vi "small_cap_hod_momentum.vi"() -> ()   [LabVIEW 2023]
panel:
  in  "MCLB":i32(listbox)
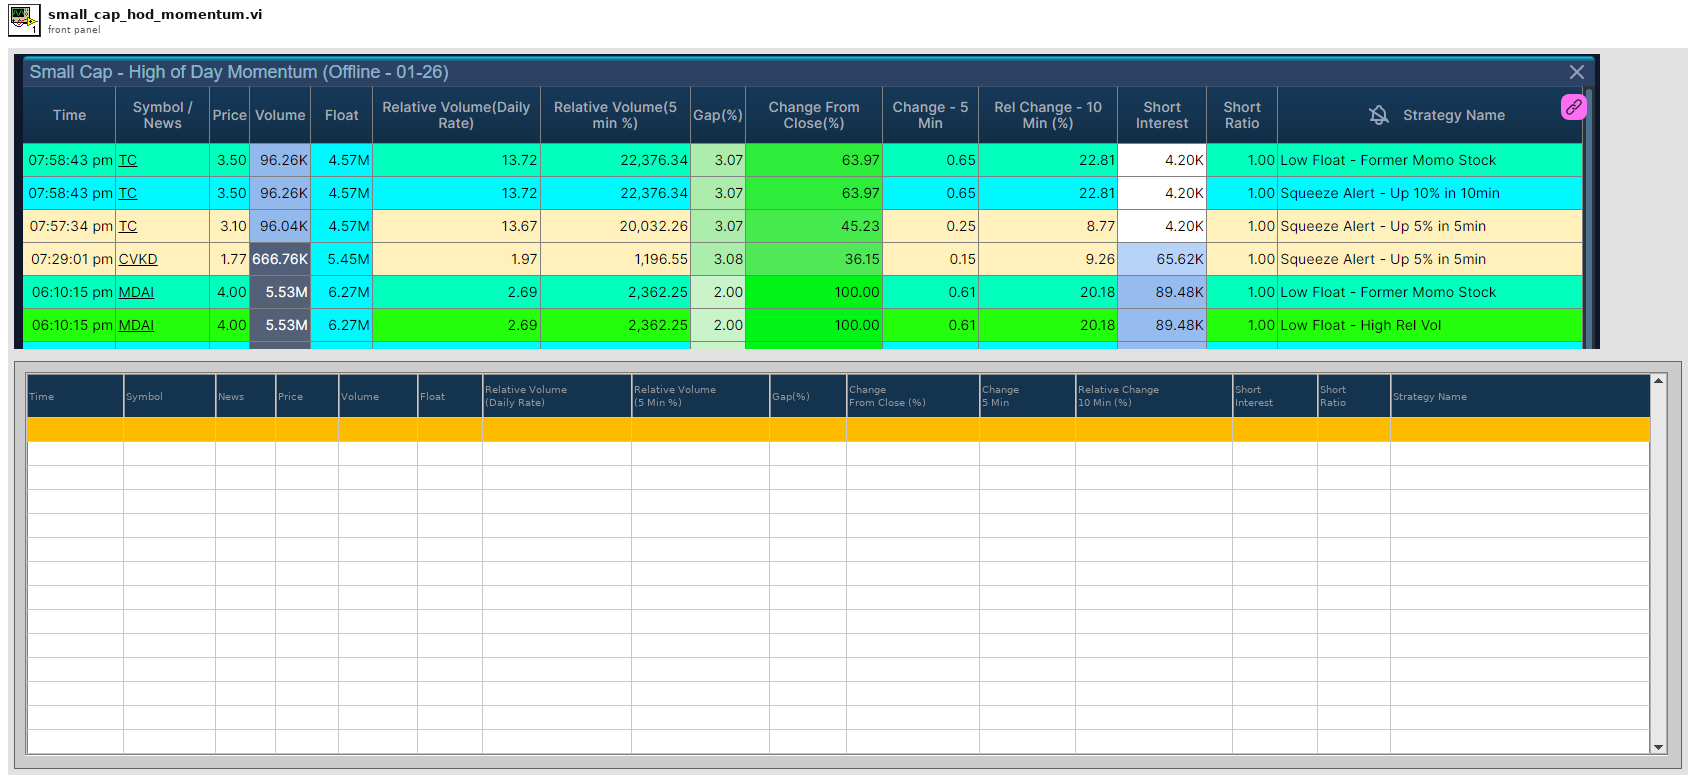
[diagram p1: front panel]
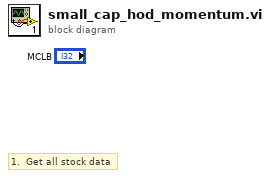
[diagram p0: block diagram]
diagram:
  # "1.  Get all stock data"
